vi "Make phase.vi"(9 "previous cycle":dbl, 10 "Time":dbl[](array[numeric]), 11 "Current treatment":T1={"sample"=0.0, "startphase"=0.0, "type"=enum."Zero", "frequency"=0.0, "amplitude"=0.0, "noise"=0.0, "duration"=inf, "kfreq"=0.0, "noisehifreq"=0.0, "frequency2"=0.0, "amplitude2"=0.0, "startphase2"=0.0, "noise filter type"=enum."Lowpass", "noiselofreq"=0.0, "amp change"=0.0, "noise change"=0.0}) -> (2 "cycle":dbl[](array[numeric]), 3 "phase":dbl[](array[numeric]))   [LabVIEW 2012]
uses:
  Treatment.ctl
  Treatment type.ctl
  <vilib>/Analysis/3filter.llb/Filter Passband Type.ctl
  <vilib>/Analysis/NI_AALBase.lvlib
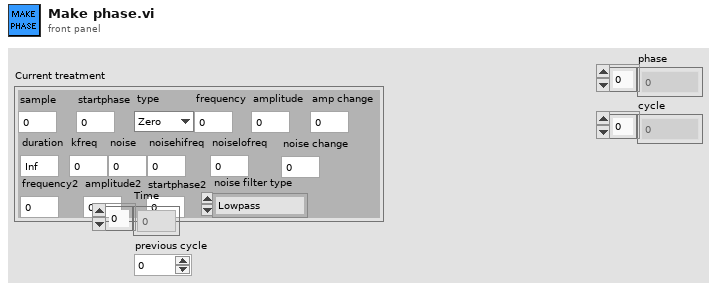
[diagram p1: front panel]
types:
  T1 = typedef "Treatment.ctl" = cluster{"sample":dbl, "startphase":dbl, "type":T2, "frequency":dbl, "amplitude":dbl, "noise":dbl, "duration":dbl, "kfreq":dbl, "noisehifreq":dbl, "frequency2":dbl, "amplitude2":dbl, "startphase2":dbl, "noise filter type":T3, "noiselofreq":dbl, "amp change":dbl, "noise change":dbl}
  T2 = typedef "Treatment type.ctl" = enum16{"Zero", "Sine", "Frequency sweep", "Two frequency", "Amplitude sweep"}
  T3 = typedef "NI_AALBase.lvlib/Filter Passband Type.ctl" = enum32{"Lowpass", "Highpass", "Bandpass", "Bandstop"}
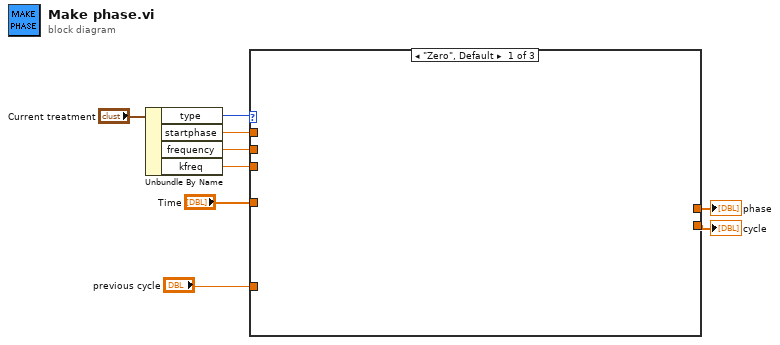
[diagram p0: block diagram]
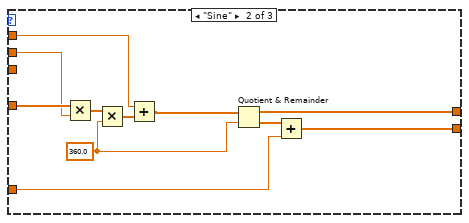
[diagram p2: hidden frame]
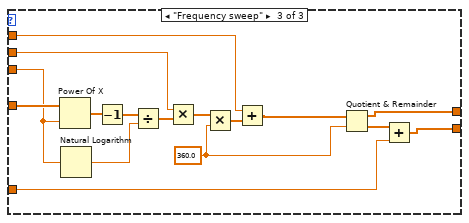
[diagram p3: hidden frame]
diagram:
  n1 = Unbundle By Name("Current treatment") -> ("type"=w8:T2, "startphase"=w5:dbl, "frequency"=w6:dbl, "kfreq"=w2:dbl)
  n2 = case shown="\"Zero\", Default" w8 {
    tunnel: "Time" -> [_ w15 w36]
    tunnel: w6 -> [_ w14 w30]
    tunnel: w5 -> [_ w13 w25]
    tunnel: "previous cycle" -> [_ w12 w23]
    tunnel: [_ w11 w22] -> w4
    tunnel: [_ w10 w21] -> w3
    tunnel: w2 -> [_ _ w34]
    frame "Zero", Default {
    }
    frame "Sine" {
      w18 = 360.0
      n3 = Multiply(x=w15, y=w14) -> (x*y=w20:dbl[])
      n4 = Multiply(x=w20, y=w18) -> (x*y=w19:dbl[])
      n5 = Add(x=w13, y=w19) -> (x+y=w16:dbl[])
      n6 = Quotient & Remainder(x=w16, y=w18) -> (x-y*floor(x/y)=w11:dbl[], floor(x/y)=w17:dbl[])
      n7 = Add(x=w17, y=w12) -> (x+y=w10:dbl[])
    }
    frame "Frequency sweep" {
      w24 = 360.0
      n8 = Power Of X(1:w34, 2:w36) -> (0:w35:dbl[])
      n9 = Natural Logarithm(1:w34) -> (0:w32:dbl)
      n10 = Decrement(x=w35) -> (x-1=w33:dbl[])
      n11 = Divide(x=w33, y=w32) -> (x/y=w31:dbl[])
      n12 = Multiply(x=w30, y=w31) -> (x*y=w26:dbl[])
      n13 = Multiply(x=w26, y=w24) -> (x*y=w29:dbl[])
      n14 = Add(x=w25, y=w29) -> (x+y=w27:dbl[])
      n15 = Quotient & Remainder(x=w27, y=w24) -> (x-y*floor(x/y)=w22:dbl[], floor(x/y)=w28:dbl[])
      n16 = Add(x=w28, y=w23) -> (x+y=w21:dbl[])
    }
  }
  "phase" <- w4
  "cycle" <- w3
